vi "Request Data JSON.vi"(8 "error in (no error)":errorcluster, 11 "GetInputVolume in":refnum<class "GetInputVolume.lvclass">) -> (0 "error out":errorcluster, 2 "Request Data JSON":string, 3 "GetInputVolume out":refnum<class "GetInputVolume.lvclass">)   [LabVIEW 2022 SP3, in "obs-websocket-lv.lvlib" / "GetInputVolume.lvclass"]
uses:
  GetInputVolume.lvclass
  GetInputVolume.lvclass/GetInputVolume.ctl
  <vilib>/IlluminatedG/lv-web-crypto/lv-json/JSON/JSON.lvlib
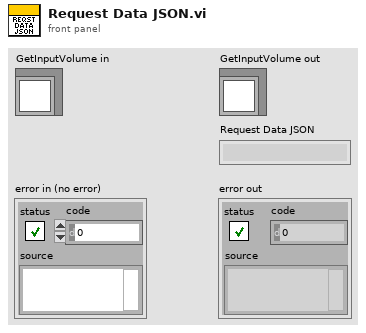
[diagram p1: front panel]
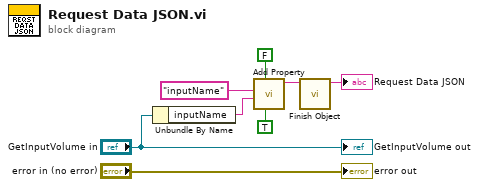
[diagram p0: block diagram]
diagram:
  n1 = Unbundle By Name("GetInputVolume in") -> ("inputName"=w3:string)
  n2 = call <vilib>:"Add Property.vi"("String?"=TRUE, "Include Empty?"=FALSE, "Value"=w3, "Property Name"="inputName") -> ("String out"=w2:string)  [unwired: 7 in]
  n3 = call <vilib>:"Finish Object.vi"("String In"=w2) -> ("String out"=→"Request Data JSON":string)  [unwired: 10 in]
  "error out" <- "error in (no error)"
  "GetInputVolume out" <- "GetInputVolume in"
